vi "SubVI1.vi"() -> ()   [LabVIEW 2013]
panel:
  out "Loop Count":i32
  in  "Stop":bool
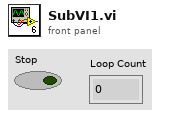
[diagram p1: front panel]
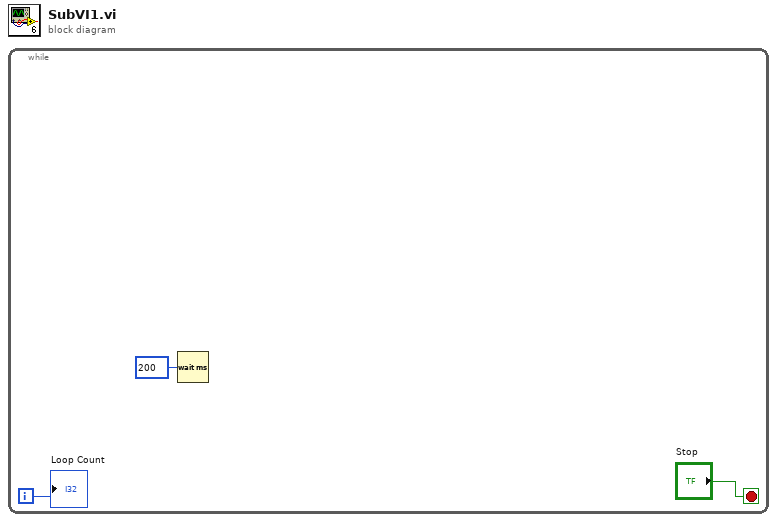
[diagram p0: block diagram]
diagram:
  n1 = while {
    i -> [w1]
    stop <- "Stop" stop-if-true
    n2 = Wait (ms)(milliseconds to wait=u32 200) -> ()  [unwired: 1 out]
    "Loop Count" <- w1
  }
